vi "Insert Into Array (Single).vi"(8 "error in (no error)":errorcluster, 9 "index":i32, 10 "JSON Datatype":refnum<class "JSON Datatype.lvclass">, 11 "JSON Array in":refnum<class "JSON Array.lvclass">) -> (0 "error out":errorcluster, 3 "JSON Array out":refnum<class "JSON Array.lvclass">)   [LabVIEW 2017, in "LVJSON.lvlib" / "JSON Array.lvclass"]
uses:
  JSON Array.lvclass
  JSON Datatype/JSON Datatype.lvclass
  JSON Array.lvclass/JSON Array.ctl
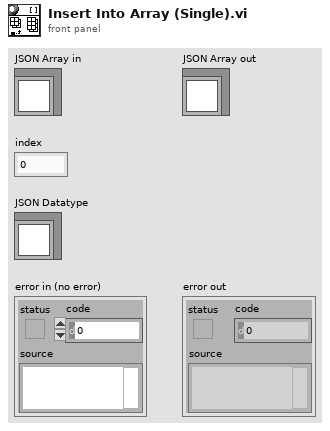
[diagram p1: front panel]
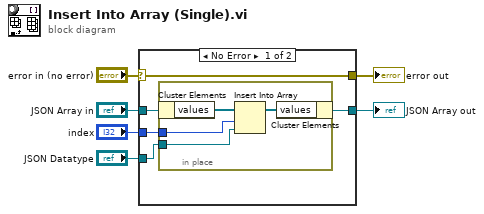
[diagram p0: block diagram]
diagram:
  n1 = case shown="No Error" "error in (no error)" {
    selector: "error in (no error)" -> [w8 w17]
    tunnel: [w8 w17] -> w5
    tunnel: [w9 w16] -> w3
    tunnel: "JSON Array in" -> [w10 w16]
    tunnel: "JSON Datatype" -> [w7 _]
    tunnel: "index" -> [w11 _]
    frame No Error {
      n2 = in-place {
        in-place-border: w7 -> [w13]
        in-place-border: w11 -> [w15]
        n3 = in-place-cluster #1(w10) -> ("values"=w12:refnum<class "JSON Datatype.lvclass">[])
        n4 = Insert Into Array(array=w12, index=w15, new element=w13) -> (w14:refnum<class "JSON Datatype.lvclass">[])
        n5 = in-place-cluster #1("values"=w14) -> (w9:refnum<class "JSON Array.lvclass">)
      }
    }
    frame Error {
    }
  }
  "error out" <- w5
  "JSON Array out" <- w3
